vi "SA40060.20210626 BG.vi"() -> ()   [LabVIEW 2020]
uses:
  <vilib>/Analysis/baseanly.llb/Mean (DBL).vi
  <userlib>/_OpenG.lib/file/file.llb/Build Path - Traditional__ogtk.vi
  <userlib>/LevyLab/LV to ITX/Data/Data.lvclass
  <userlib>/LevyLab/XY Utilities/xy_utilities.lvlib
  <vilib>/Analysis/NI_AALBase.lvlib
panel:
  in  "Temps to keep (Lifespan)":i32=26
  out "Lifespan vs Temp (hrs)":cluster{i32[], dbl[]}[](graph)
  out "E_a":dbl[](array[numeric])
  out "Arrhenius":T1(graph)
  in  "Temps to keep (Arrhenius fit)":i32=26
  out "G2T vs t BG":T1(graph)
  out "G4T vs t BG":T1(graph)
  out "Temp vs t":T1(graph)
  in  "Source Voltage":dbl=0.1
  in  "Init Temp":i32=275
  in  "Temp Step":i32=5
  in  "Final Temp":i32=400
  in  "Data File":path=path "G:/My Drive/ansom/Data/PPMS 2/SA40060.20210626/00 - BG ONLY/SA40060.20210626.275K.dat"
  in  "Trimming":i32=400
  in  "Update":bool
  in  "OK":bool
  out "error out":errorcluster
  in  "error in (no error)":errorcluster
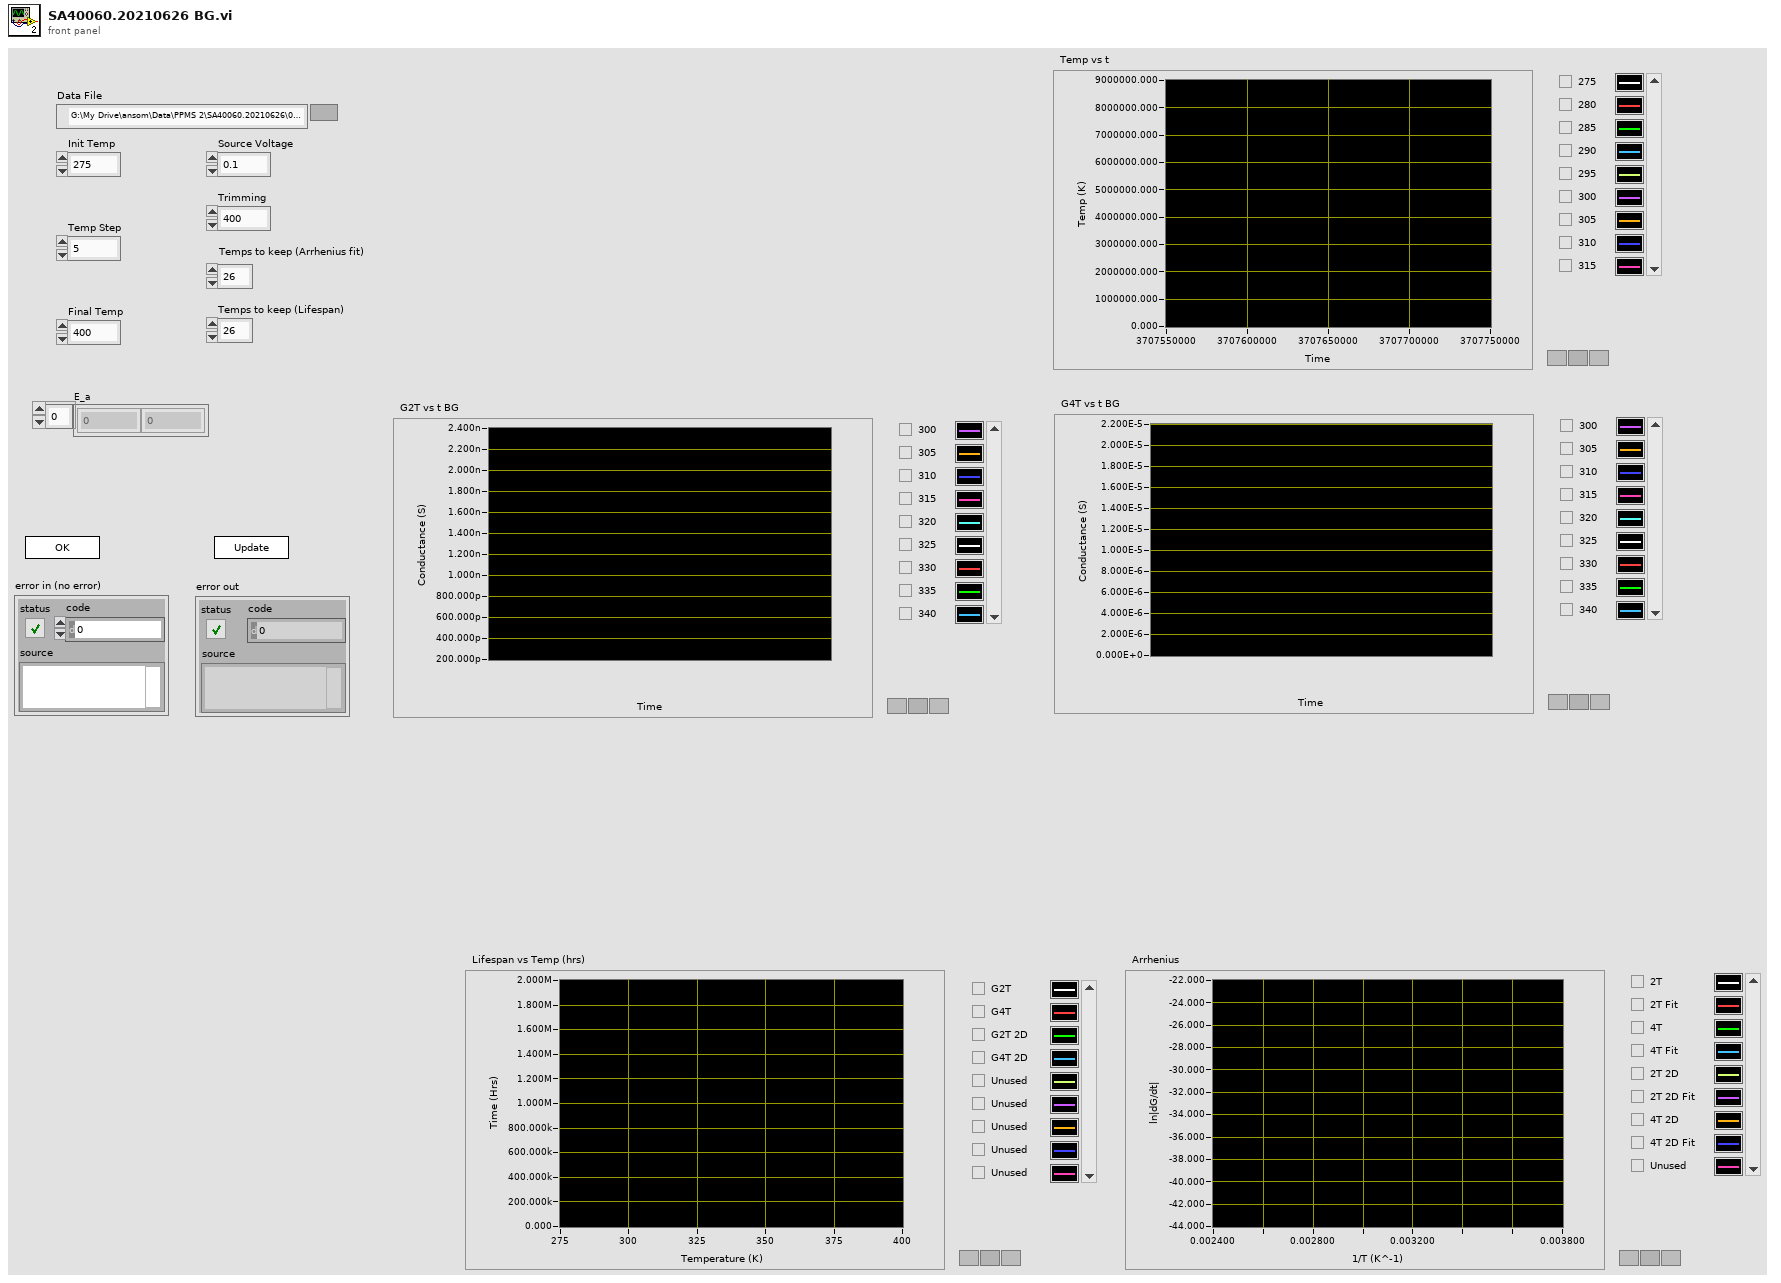
[diagram p1: front panel]
types:
  T1 = cluster{"Data":dbl[], "Best Exponential Fit":dbl[]}[]
  T2 = enum32{"Invalid", "Standard", "Closed", "Hidden", "Minimized", "Maximized"}
  T3 = enum32{"invalid app kind", "Development System", "Run Time System", "Student Edition", "Embedded LabVIEW", "Evaluation", "Custom"}
  T4 = cluster{"Core":cluster{"Current VI Reference":refnum<vi>, "Close Panel on Exit?":bool}, "G2T 1D":cluster{dbl[], dbl[]}[], "G4T 1D":cluster{dbl[], dbl[]}[], "Temp":cluster{dbl[], dbl[]}[], "Source Voltage":dbl, "Final Temp":i32, "Init Temp":i32, "Temp Step":i32, "Data File":path, "Trimming":i32}
  T5 = cluster{"Current VI Reference":refnum<vi>, "Close Panel on Exit?":bool}
  T6 = typedef "Data.lvclass/Dictionary--cluster.ctl" = cluster{"key":string, "value":variant}
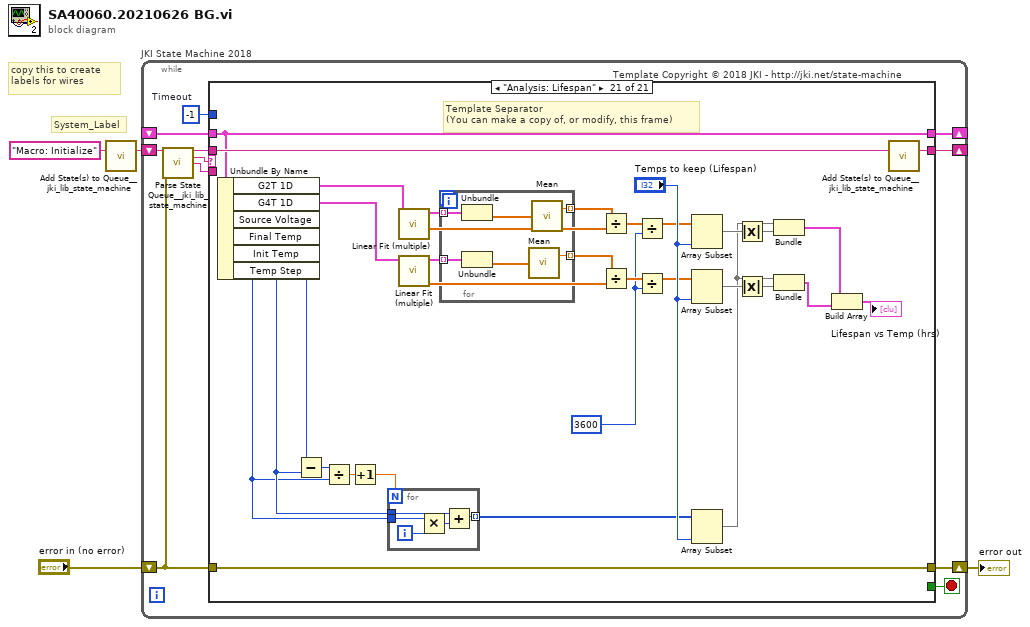
[diagram p0: block diagram]
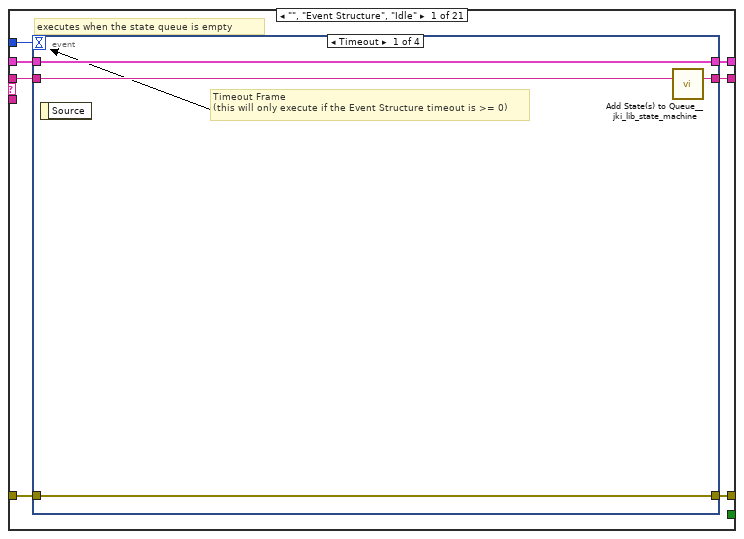
[diagram p2: hidden frame]
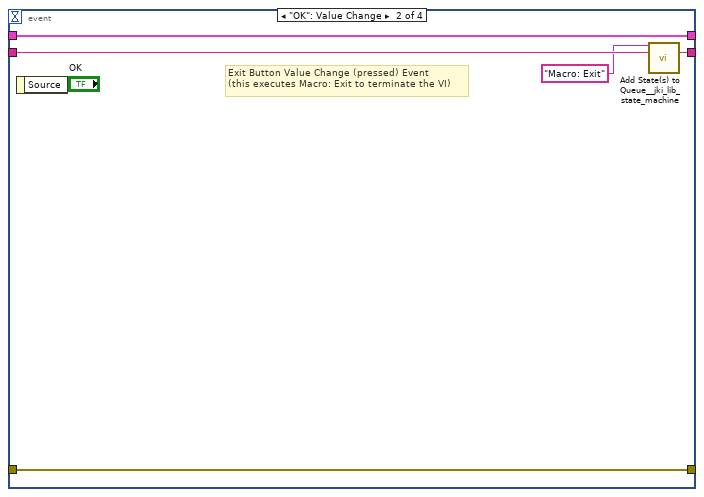
[diagram p3: hidden frame]
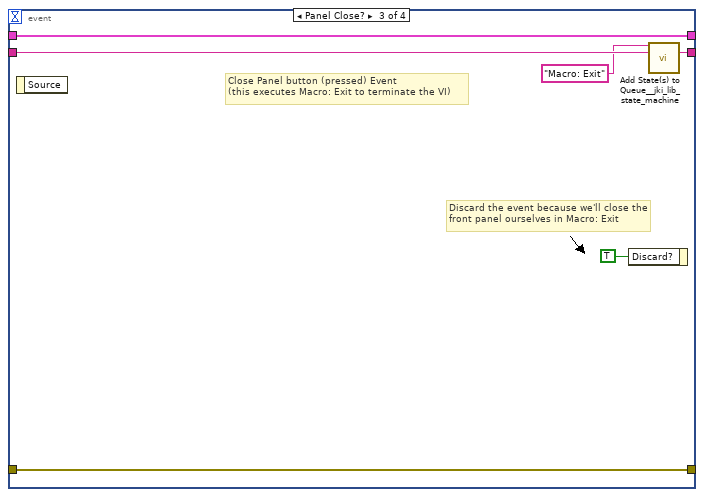
[diagram p4: hidden frame]
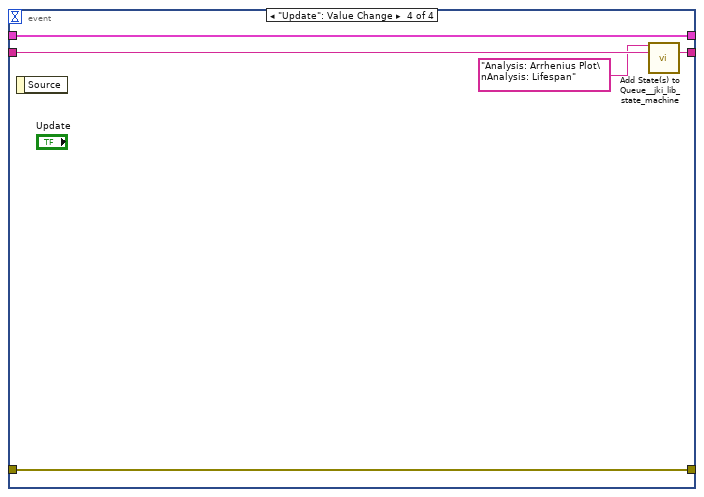
[diagram p5: hidden frame]
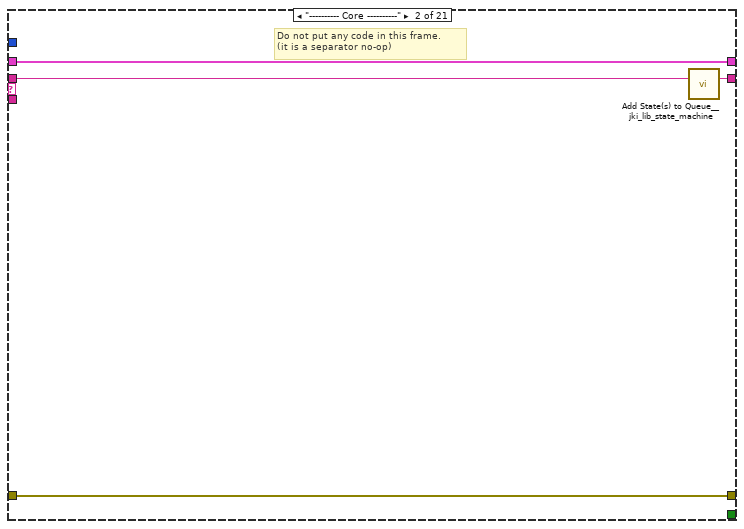
[diagram p6: hidden frame]
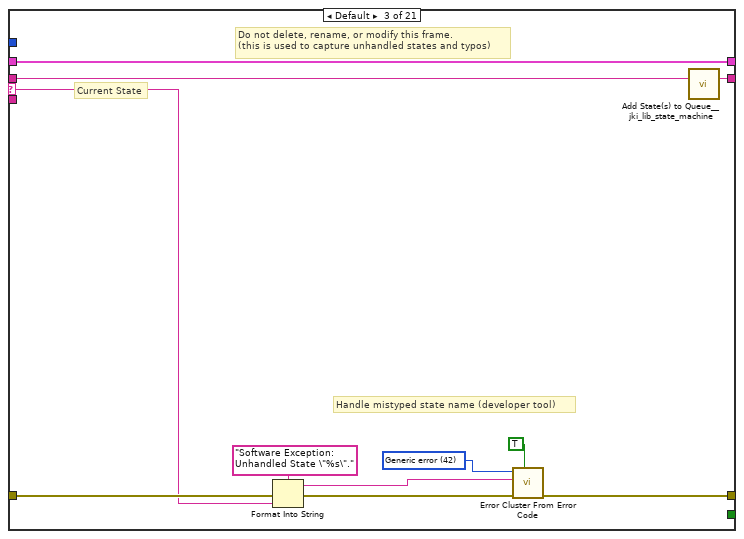
[diagram p7: hidden frame]
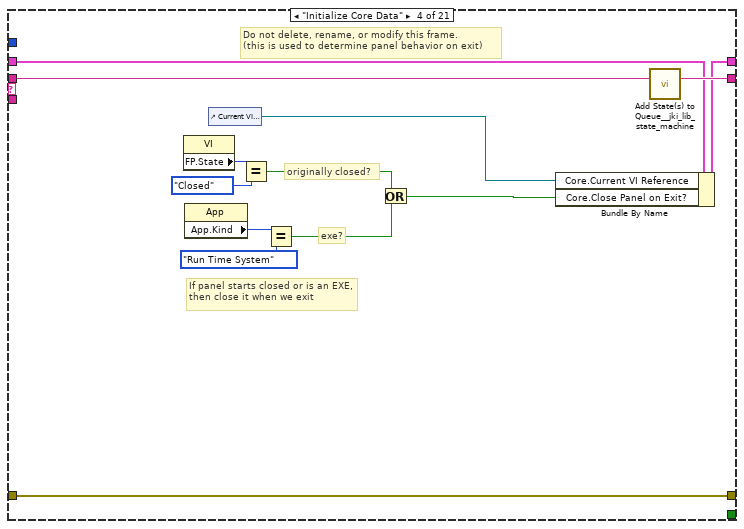
[diagram p8: hidden frame]
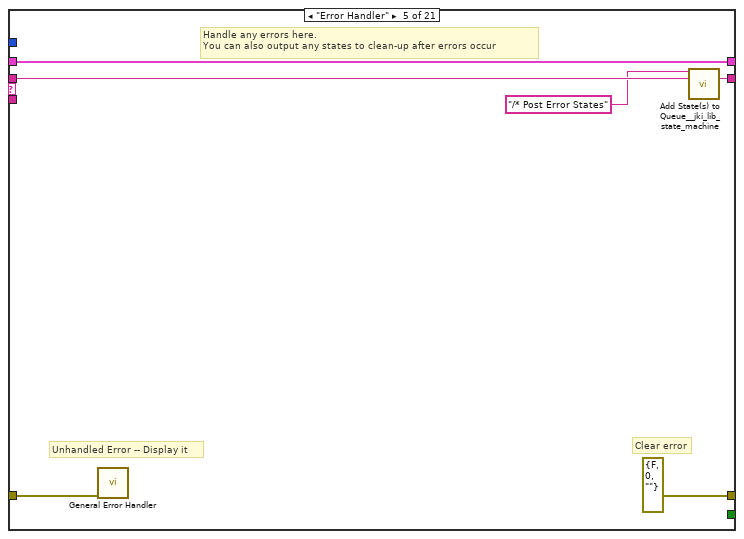
[diagram p9: hidden frame]
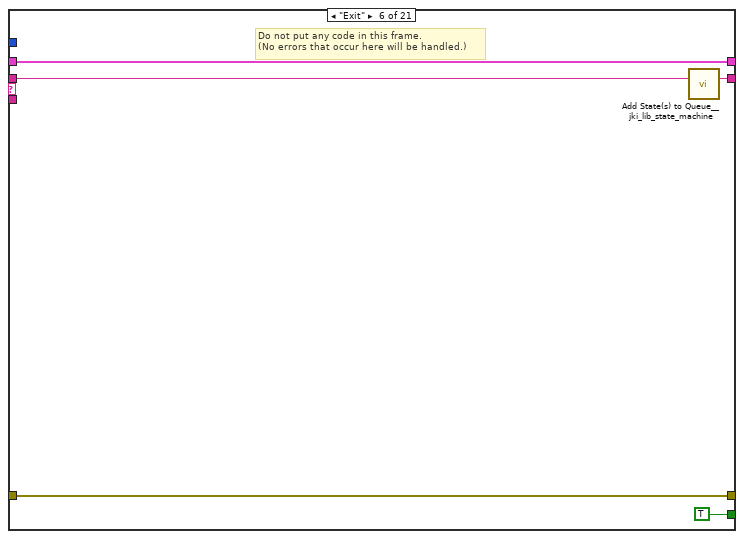
[diagram p10: hidden frame]
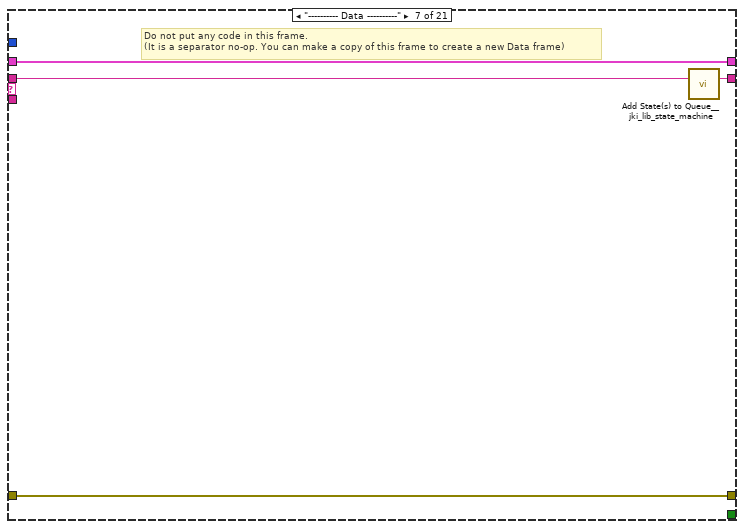
[diagram p11: hidden frame]
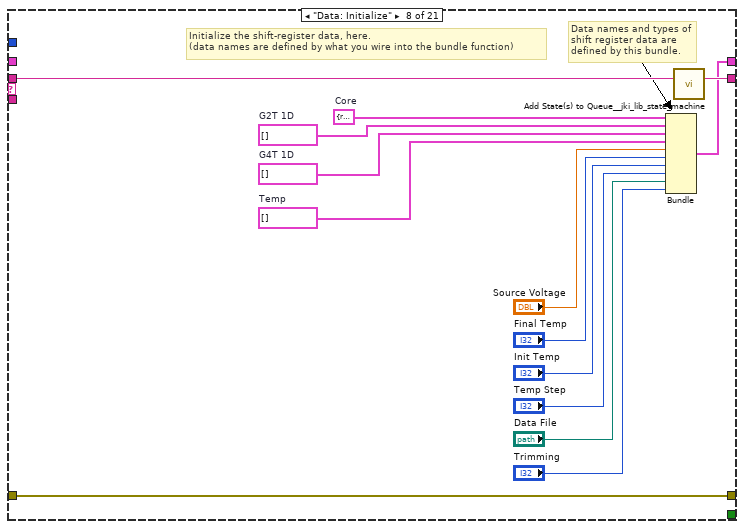
[diagram p12: hidden frame]
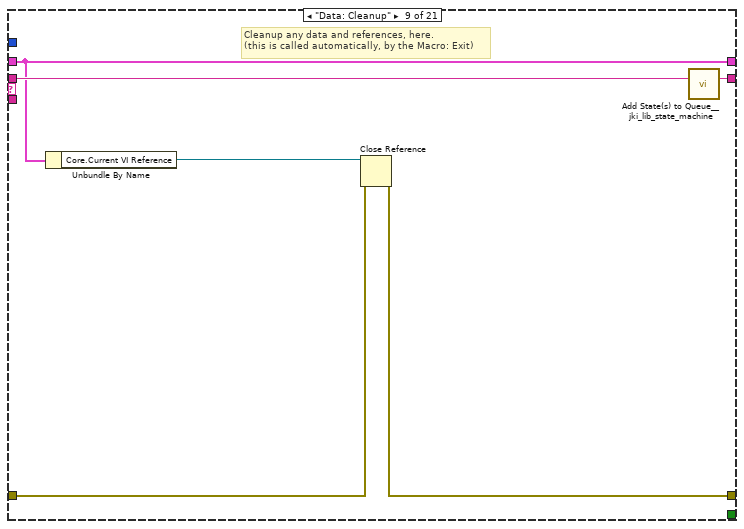
[diagram p13: hidden frame]
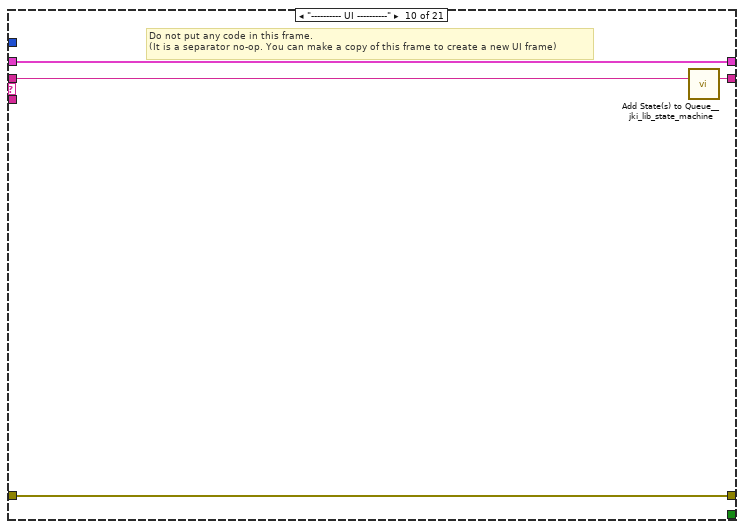
[diagram p14: hidden frame]
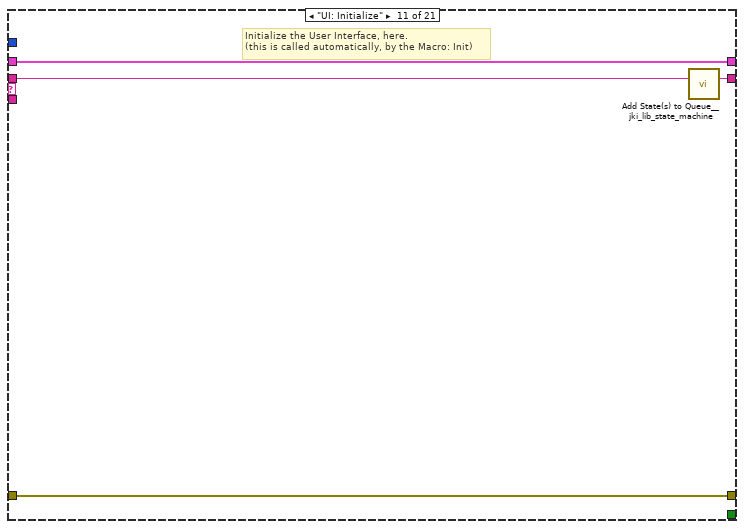
[diagram p15: hidden frame]
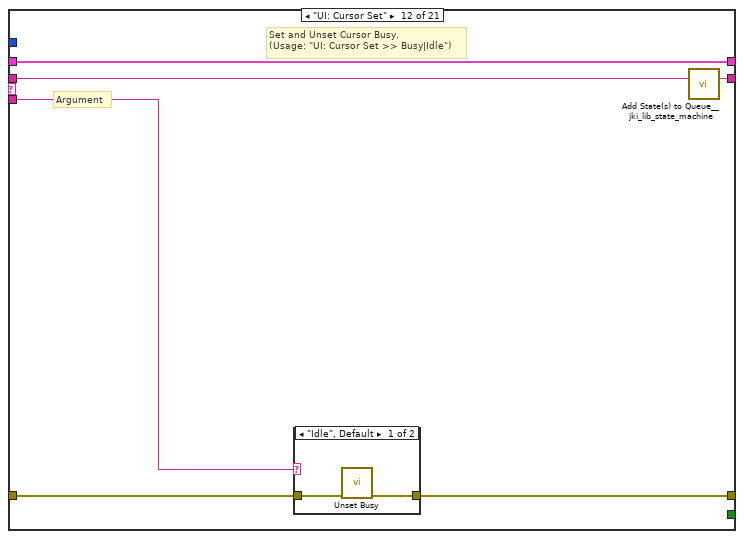
[diagram p16: hidden frame]
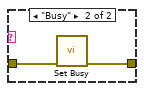
[diagram p17: hidden frame]
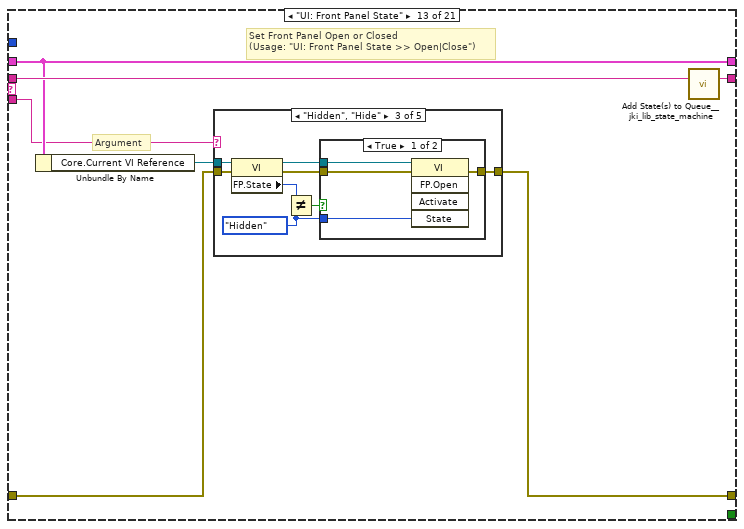
[diagram p18: hidden frame]
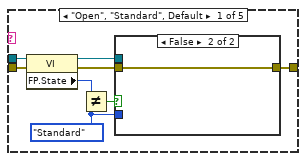
[diagram p19: hidden frame]
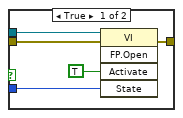
[diagram p20: hidden frame]
diagram:
  # "copy this to create labels for wires"
  # "System_Label"
  n1 = call <vilib>:"Add State(s) to Queue__jki_lib_state_machine.vi"("State(s) in (\"\")"="Macro: Initialize") -> ("States Out"=w4:string)  [unwired: 14 in]
  n2 = while "JKI State Machine 2018" {
    shift-right: [w8] -> _
    shift-left: _ -> [w7]
    shift-right: [w11] -> w1
    shift-left: "error in (no error)" -> [w5]
    shift-right: [w10] -> _
    shift-left: w4 -> [w12]
    stop <- w9 stop-if-true
    w6 = -1  # Timeout
    # "Template Copyright © 2018 JKI - http://jki.net/state-machine"
    n3 = call <vilib>:"Parse State Queue__jki_lib_state_machine.vi"("State Queue"=w12, "Error In (no error)"=w5) -> ("Remaining States"=w14:string, "Current State"=w15:string, "Arguments"=w13:string)  [unwired: 11 in]
    n4 = case shown="\"Analysis: Lifespan\"" w15 {
      selector: w15 -> [_ _ w47 _ _ _ _ _ _ _ _ _ _ _ _ _ _ _ _ _ _]
      tunnel: w14 -> [w22 w46 w51 w70 w76 w81 w85 w99 w105 w109 w113 w119 w130 w199 w204 w214 w218 w235 w282 w314 w353]
      tunnel: w13 -> [_ _ _ _ _ _ _ _ _ _ _ w114 w124 _ _ _ _ _ _ _ _]
      tunnel: w7 -> [w20 w43 w49 w63 w73 w79 w82 _ w100 w106 w111 w117 w126 w196 w201 w211 w215 w229 w279 w311 w339]
      tunnel: [w19 w44 w53 w67 errorcluster {"status"=FALSE, "code"=0, "source"=""} ("error out") w78 w83 w96 w101 w107 w110 w115 w127 w197 w202 w212 w216 w231 w280 w312 w351] -> w11
      tunnel: w5 -> [w18 w44 w52 w67 w72 w78 w83 w96 w102 w107 w110 w116 w128 w197 w202 w212 w216 w231 w280 w312 w351]
      tunnel: [w21 w45 w50 w69 w75 w80 w84 w98 w104 w108 w112 w118 w129 w198 w203 w213 w217 w234 w281 w313 w352] -> w10
      tunnel: [_ _ _ _ _ TRUE _ _ _ _ _ _ _ _ _ _ _ _ _ _ _] -> w9
      tunnel: [w17 w43 w49 w68 w73 w79 w82 w97 w100 w106 w111 w117 w126 w196 w201 w211 w215 w230 w279 w311 w339] -> w8
      tunnel: w6 -> [w16 _ _ _ _ _ _ _ _ _ _ _ _ _ _ _ _ _ _ _ _]
      frame "", "Event Structure", "Idle" {
        # "executes when the state queue is empty"
        n5 = event shown="[0] Timeout" {
          selector: _ -> [_ _ _ _]
          dyn-events: _ -> [_ _ _ _]
          timeout: w16 -> [_ _ _ _]
          tunnel: w22 -> [w26 w31 w37 w41]
          tunnel: [w25 w30 w36 w40] -> w21
          tunnel: w20 -> [w23 w28 w34 w42]
          tunnel: [w24 w29 w35 w38] -> w19
          tunnel: w18 -> [w24 w29 w35 w38]
          tunnel: [w23 w28 w34 w42] -> w17
          event Timeout {
            # "Timeout Frame\n(this will only execute if the Event Structure timeout is >= 0)"
            n6 = event-data() -> ()  [unwired: 1 in, 1 out]
            n7 = call <vilib>:"Add State(s) to Queue__jki_lib_state_machine.vi"("State(s) in (\"\")"=w26) -> ("States Out"=w25:string)  [unwired: 14 in]
          }
          event "OK": Value Change {
            # "Exit Button Value Change (pressed) Event\n(this executes Macro: Exit to terminate the VI)"
            n8 = event-data() -> ()  [unwired: 1 in, 1 out]
            n9 = call <vilib>:"Add State(s) to Queue__jki_lib_state_machine.vi"("State(s) in Front (\"\")"="Macro: Exit", "State(s) in (\"\")"=w31) -> ("States Out"=w30:string)  [unwired: 13 in]
          }
          event Panel Close? {
            # "Discard the event because we'll close the front panel ourselves in Macro: Exit"
            # "Close Panel button (pressed) Event\n(this executes Macro: Exit to terminate the VI)"
            n10 = event-data() -> ()  [unwired: 1 in, 1 out]
            n11 = event-data("Discard?"=TRUE) -> ()  [unwired: 1 in, 1 out]
            n12 = call <vilib>:"Add State(s) to Queue__jki_lib_state_machine.vi"("State(s) in Front (\"\")"="Macro: Exit", "State(s) in (\"\")"=w37) -> ("States Out"=w36:string)  [unwired: 13 in]
          }
          event "Update": Value Change {
            n13 = event-data() -> ()  [unwired: 1 in, 1 out]
            n14 = call <vilib>:"Add State(s) to Queue__jki_lib_state_machine.vi"("State(s) in Front (\"\")"="Analysis: Arrhenius Plot\nAnalysis: Lifespan" ("State(s) in Front (\"\")"), "State(s) in (\"\")"=w41) -> ("States Out"=w40:string)  [unwired: 13 in]
          }
        }
      }
      frame "---------- Core ----------" {
        # "Do not put any code in this frame.\n(it is a separator no-op)"
        n15 = call <vilib>:"Add State(s) to Queue__jki_lib_state_machine.vi"("State(s) in (\"\")"=w46) -> ("States Out"=w45:string)  [unwired: 14 in]
      }
      frame Default {
        w56 = 42 items=["No error", "Argument error", "Memory is full", "Out of zone", "End of file", "File already open", "Generic file I/O error", "File not found", "File permission error", "Disk is full", "Duplicate path", "Too many files open", "System feature not enabled", "Resource file not found", "Cannot add resource", "Resource not found", "Image not found", "Image memory error", "Pen does not exist", "Config type invalid", "Config token not found", "Config parse error", "Config memory error", "Bad external code format", "Bad external code offset", "External code not present", "Null window", "Destroy window error", "Null menu", "Print aborted", "Bad print record", "Print driver error", "Windows error during printing", "Memory error during printing", "Print dialog error", "Generic print error", "Invalid device refnum", "Device not found", "Device parameter error", "Device unit error", "Cannot open device", "Device call aborted", "Generic error", "Cancelled by user", "Object ID too low", "Object ID too high", "Object not in heap", "Unknown heap", "Unknown object (invalid DefProc)", "Unknown object (DefProc not in table)", "Message out of range", "Invalid (null) method", "Unknown message", "Manager call not supported", "Bad address", "Network operation in progress", "Network operation timed out", "Connection is busy", "Network attribute not supported", "Network error", "Address in use", "System out of memory", "Connection aborted", "Connection refused", "Not connected", "Already connected", "Connection closed", "Initialization error (interapplication manager)", "Bad occurrence", "Wait on unbound occurrence handler", "Occurrence queue overflow", "Datalog type conflict", "Unused", "Unrecognized type (interapplication manager)", "Memory corrupt", "Failed to make temporary DLL", "Old CIN version", "Drag socket not found", "Failed to load drop-object", "Failed to register OLE object", "Failed to release OLE object", "Format specifier type mismatch", "Unknown format specifier", "Too few format specifiers", "Too many format specifiers", "Scan failed", "Newer CIN version", "Error converting to variant", "Runtime menu error", "Password tampered", "Variant attribute not found", "Incompatible variant data type", "Event data is not available", "Event Store is not present", "Occurrence is not found", "Event Queue is not created", "Event info is not available", "Refnum passed is NULL", "Error retrieving Class GUID", "Error retrieving CoClass GUID", "Error retrieving TypeLib GUID.", "Bad built application magic bytes.", "Specific driver is different from the specific driver associated with the Logical Name.", "There is no session opened to the class driver.", "Max Error", "MAX - Error with config objects", "MAX - Error loading configuration", "MAX - Group not supported"]
        # "Current State"
        # "Do not delete, rename, or modify this frame.\n(this is used to capture unhandled states and typos)"
        # "Handle mistyped state name (developer tool)"
        n16 = Format Into String(format string="Software Exception: Unhandled State \"%s\"." ("message"), error in=w52, w47) -> (resulting string=w55:string, error out=w54:errorcluster)  [unwired: 1 in]
        n17 = call <vilib>:"Error Cluster From Error Code.vi"("show call chain? (False)"=TRUE, "error in (no error)"=w54, "error message (\"\")"=w55, "error code (0)"=w56) -> ("error out"=w53:errorcluster)  [unwired: 5 in]
        n18 = call <vilib>:"Add State(s) to Queue__jki_lib_state_machine.vi"("State(s) in (\"\")"=w51) -> ("States Out"=w50:string)  [unwired: 14 in]
      }
      frame "Initialize Core Data" {
        # "Do not delete, rename, or modify this frame.\n(this is used to determine panel behavior on exit)"
        # "originally closed?"
        # "exe?"
        # "If panel starts closed or is an EXE, then close it when we exit"
        n19 = property class="VI"() -> ("FP.State"=w60:T2)  [unwired: 2 in, 2 out]
        n20 = property class="App"() -> ("App.Kind"=w66:T3)  [unwired: 2 in, 2 out]
        n21 = control-ref of="Current VI Reference"() -> (w61:refnum<vi>)
        n22 = Equal?(x=w60, y=T2."Closed" ("Front Panel Window:State")) -> (x = y?=w58:bool)
        n23 = Equal?(x=w66, y=T3."Run Time System" ("Application:Kind")) -> (x = y?=w64:bool)
        n24 = Or(x=w58, y=w64) -> (x .or. y?=w62:bool)
        n25 = Bundle By Name(cluster=w63, "Core.Current VI Reference"=w61, "Core.Close Panel on Exit?"=w62) -> (w68:T4)
        n26 = call <vilib>:"Add State(s) to Queue__jki_lib_state_machine.vi"("State(s) in (\"\")"=w70) -> ("States Out"=w69:string)  [unwired: 14 in]
      }
      frame "Error Handler" {
        # "Unhandled Error -- Display it"
        # "Handle any errors here.\nYou can also output any states to clean-up after errors occur"
        # "Clear error"
        n27 = call <vilib>:"General Error Handler.vi"("error in (no error)"=w72) -> ()  [unwired: 10 in, 5 out]
        n28 = call <vilib>:"Add State(s) to Queue__jki_lib_state_machine.vi"("State(s) in Front (\"\")"="/* Post Error States", "State(s) in (\"\")"=w76) -> ("States Out"=w75:string)  [unwired: 13 in]
      }
      frame "Exit" {
        # "Do not put any code in this frame.\n(No errors that occur here will be handled.)"
        n29 = call <vilib>:"Add State(s) to Queue__jki_lib_state_machine.vi"("State(s) in (\"\")"=w81) -> ("States Out"=w80:string)  [unwired: 14 in]
      }
      frame "---------- Data ----------" {
        # "Do not put any code in this frame.\n(It is a separator no-op. You can make a copy of this frame to create a new Data frame)"
        n30 = call <vilib>:"Add State(s) to Queue__jki_lib_state_machine.vi"("State(s) in (\"\")"=w85) -> ("States Out"=w84:string)  [unwired: 14 in]
      }
      frame "Data: Initialize" {
        w86 = cluster{dbl[], dbl[]}[] []  # Temp
        w93 = cluster{dbl[], dbl[]}[] []  # G4T 1D
        w92 = cluster{dbl[], dbl[]}[] []  # G2T 1D
        w95 = T5 {"Current VI Reference"=refnum, "Close Panel on Exit?"=FALSE}  # Core
        # "Data names and types of shift register data are defined by this bundle."
        # "Initialize the shift-register data, here.\n(data names are defined by what you wire into the bundle function)"
        n31 = Bundle("Core"=w95, "G2T 1D"=w92, "G4T 1D"=w93, "Temp"=w86, "Source Voltage"="Source Voltage", "Final Temp"="Final Temp", "Init Temp"="Init Temp", "Temp Step"="Temp Step", "Data File"="Data File", "Trimming"="Trimming") -> (w97:T4)  [unwired: 1 in]
        n32 = call <vilib>:"Add State(s) to Queue__jki_lib_state_machine.vi"("State(s) in (\"\")"=w99) -> ("States Out"=w98:string)  [unwired: 14 in]
      }
      frame "Data: Cleanup" {
        # "Cleanup any data and references, here.\n(this is called automatically, by the Macro: Exit)"
        n33 = Unbundle By Name(w100) -> ("Core.Current VI Reference"=w103:refnum<vi>)
        n34 = Close Reference(reference=w103, error in (no error)=w102) -> (error out=w101:errorcluster)
        n35 = call <vilib>:"Add State(s) to Queue__jki_lib_state_machine.vi"("State(s) in (\"\")"=w105) -> ("States Out"=w104:string)  [unwired: 14 in]
      }
      frame "---------- UI ----------" {
        # "Do not put any code in this frame.\n(It is a separator no-op. You can make a copy of this frame to create a new UI frame)"
        n36 = call <vilib>:"Add State(s) to Queue__jki_lib_state_machine.vi"("State(s) in (\"\")"=w109) -> ("States Out"=w108:string)  [unwired: 14 in]
      }
      frame "UI: Initialize" {
        # "Initialize the User Interface, here.\n(this is called automatically, by the Macro: Init)"
        n37 = call <vilib>:"Add State(s) to Queue__jki_lib_state_machine.vi"("State(s) in (\"\")"=w113) -> ("States Out"=w112:string)  [unwired: 14 in]
      }
      frame "UI: Cursor Set" {
        # "Argument"
        # "Set and Unset Cursor Busy.\n(Usage: \"UI: Cursor Set >> Busy|Idle\")"
        n38 = case shown="\"Idle\", Default" w114 {
          tunnel: w116 -> [w121 w123]
          tunnel: [w120 w122] -> w115
          frame "Idle", Default {
            n39 = call <vilib>:"Unset Busy.vi"("error in (no error)"=w121) -> ("error out"=w120:errorcluster)  [unwired: 10 in]
          }
          frame "Busy" {
            n40 = call <vilib>:"Set Busy.vi"("error in (no error)"=w123) -> ("error out"=w122:errorcluster)  [unwired: 9 in, 1 out]
          }
        }
        n41 = call <vilib>:"Add State(s) to Queue__jki_lib_state_machine.vi"("State(s) in (\"\")"=w119) -> ("States Out"=w118:string)  [unwired: 14 in]
      }
      frame "UI: Front Panel State" {
        # "Argument"
        # "Set Front Panel Open or Closed\n(Usage: \"UI: Front Panel State >> Open|Close\")"
        n42 = Unbundle By Name(w126) -> ("Core.Current VI Reference"=w125:refnum<vi>)
        n43 = case shown="\"Hidden\", \"Hide\"" w124 {
          tunnel: w128 -> [w136 w151 w162 w175 w188]
          tunnel: [w138 w152 w164 w177 w190] -> w127
          tunnel: w125 -> [w137 w149 w163 w176 w189]
          frame "Open", "Standard", Default {
            w131 = T2."Standard" ("State")
            n44 = property class="VI"(reference=w137, error in=w136) -> (reference out=w134:refnum<vi>, error out=w135:errorcluster, "FP.State"=w133:T2)
            n45 = Not Equal?(x=w133, y=w131) -> (x != y?=w132:bool)
            n46 = case shown="False" w132 {
              tunnel: [w142 w144] -> w138
              tunnel: w135 -> [w141 w144]
              tunnel: w134 -> [w140 _]
              tunnel: w131 -> [w139 _]
              frame True {
                n47 = invoke class="VI" method="FP.Open"(reference=w140, error in=w141, "Activate"=TRUE, "State"=w139) -> (error out=w142:errorcluster)  [unwired: 1 in, 4 out]
              }
              frame False {
              }
            }
          }
          frame "Close", "Closed" {
            n48 = property class="VI"(reference=w149, error in=w151) -> (reference out=w148:refnum<vi>, error out=w150:errorcluster, "FP.State"=w146:T2)
            n49 = Not Equal?(x=w146, y=T2."Closed" ("Front Panel Window:State")) -> (x != y?=w145:bool)
            n50 = case shown="True" w145 {
              tunnel: [w153 w156] -> w152
              tunnel: w150 -> [w153 w155]
              tunnel: w148 -> [_ w154]
              frame False {
              }
              frame True {
                n51 = invoke class="VI" method="FP.Close"(reference=w154, error in=w155) -> (error out=w156:errorcluster)  [unwired: 1 in, 2 out]
              }
            }
          }
          frame "Hidden", "Hide" {
            w157 = T2."Hidden" ("State")
            n52 = property class="VI"(reference=w163, error in=w162) -> (reference out=w160:refnum<vi>, error out=w161:errorcluster, "FP.State"=w159:T2)
            n53 = Not Equal?(x=w159, y=w157) -> (x != y?=w158:bool)
            n54 = case shown="True" w158 {
              tunnel: [w168 w169] -> w164
              tunnel: w161 -> [w167 w169]
              tunnel: w160 -> [w166 _]
              tunnel: w157 -> [w165 _]
              frame True {
                n55 = invoke class="VI" method="FP.Open"(reference=w166, error in=w167, "State"=w165) -> (error out=w168:errorcluster)  [unwired: 2 in, 4 out]
              }
              frame False {
              }
            }
          }
          frame "Minimize", "Minimized" {
            w170 = T2."Minimized" ("State")
            n56 = property class="VI"(reference=w176, error in=w175) -> (reference out=w173:refnum<vi>, error out=w174:errorcluster, "FP.State"=w172:T2)
            n57 = Not Equal?(x=w172, y=w170) -> (x != y?=w171:bool)
            n58 = case shown="True" w171 {
              tunnel: [w181 w182] -> w177
              tunnel: w174 -> [w180 w182]
              tunnel: w173 -> [w179 _]
              tunnel: w170 -> [w178 _]
              frame True {
                n59 = invoke class="VI" method="FP.Open"(reference=w179, error in=w180, "State"=w178) -> (error out=w181:errorcluster)  [unwired: 2 in, 4 out]
              }
              frame False {
              }
            }
          }
          frame "Maximize", "Maximized" {
            w183 = T2."Maximized" ("State")
            n60 = property class="VI"(reference=w189, error in=w188) -> (reference out=w186:refnum<vi>, error out=w187:errorcluster, "FP.State"=w185:T2)
            n61 = Not Equal?(x=w185, y=w183) -> (x != y?=w184:bool)
            n62 = case shown="True" w184 {
              tunnel: [w194 w195] -> w190
              tunnel: w187 -> [w193 w195]
              tunnel: w186 -> [w192 _]
              tunnel: w183 -> [w191 _]
              frame True {
                n63 = invoke class="VI" method="FP.Open"(reference=w192, error in=w193, "State"=w191) -> (error out=w194:errorcluster)  [unwired: 2 in, 4 out]
              }
              frame False {
              }
            }
          }
        }
        n64 = call <vilib>:"Add State(s) to Queue__jki_lib_state_machine.vi"("State(s) in (\"\")"=w130) -> ("States Out"=w129:string)  [unwired: 14 in]
      }
      frame "---------- Macro ----------" {
        # "Do not put any code in this frame.\n(It is a separator no-op. You can make a copy of this frame to create a new Macro frame)"
        n65 = call <vilib>:"Add State(s) to Queue__jki_lib_state_machine.vi"("State(s) in (\"\")"=w199) -> ("States Out"=w198:string)  [unwired: 14 in]
      }
      frame "Macro: Initialize" {
        # "Initialization Macro\n(This is called once, when the VI starts)"
        n66 = call <vilib>:"Add State(s) to Queue__jki_lib_state_machine.vi"("State(s) in Front (\"\")"="Data: Initialize\nInitialize Core Data\nUI: Initialize\nUI: Front Panel State >> Open\nAnalysis: Load Data\nAnalysis: Plot G vs t\nAnalysis: Arrhenius Plot\nAnalysis: Lifespan", "State(s) in (\"\")"=w204) -> ("States Out"=w203:string)  [unwired: 13 in]
      }
      frame "Macro: Exit" {
        # "Exit Macro\n(This is called once, when the VI exits)"
        n67 = Unbundle By Name(w211) -> ("Core.Close Panel on Exit?"=w210:bool)
        n68 = Select(t="UI: Front Panel State >> Close", s=w210, f="") -> (s? t:f=w207:string)
        n69 = call <vilib>:"Add State(s) to Queue__jki_lib_state_machine.vi"("State(s) in (\"\")"=w207, "State(s) at Back (\"\")"="Data: Cleanup\nExit") -> ("States Out"=w205:string)  [unwired: 13 in]
        n70 = call <vilib>:"Add State(s) to Queue__jki_lib_state_machine.vi"("State(s) in Front (\"\")"=w205, "State(s) in (\"\")"=w214) -> ("States Out"=w213:string)  [unwired: 13 in]
      }
      frame "---------- Analysis ----------" {
        # "Template Separator\n(You can make a copy of, or modify, this frame)"
        n71 = call <vilib>:"Add State(s) to Queue__jki_lib_state_machine.vi"("State(s) in (\"\")"=w218) -> ("States Out"=w217:string)  [unwired: 14 in]
      }
      frame "Analysis: Load Data" {
        n72 = Unbundle By Name(w229) -> ("Source Voltage"=w228:dbl, "Final Temp"=w225:i32, "Init Temp"=w222:i32, "Temp Step"=w221:i32, "Data File"=w223:path, "Trimming"=w220:i32)
        n73 = Subtract(x=w225, y=w222) -> (x-y=w232:i32)
        n74 = Divide(x=w232, y=w221) -> (x/y=w233:dbl)
        n75 = Increment(x=w233) -> (x+1=w224:dbl)
        n76 = for {
          N: w224 -> [_]
          tunnel: w228 -> [w246]
          tunnel: [w263] -> w227 mode=indexing
          tunnel: [w262] -> w226 mode=indexing
          tunnel: w223 -> [w261]
          tunnel: w222 -> [w260]
          tunnel: w221 -> [w259]
          tunnel: w220 -> [w258]
          tunnel: [w255] -> w219 mode=indexing
          i -> [w266]
          n77 = Strip Path(path=w261) -> (stripped path=w271:path, name=w270:string)
          n78 = Multiply(x=w259, y=w266) -> (x*y=w267:i32)
          n79 = Add(x=w260, y=w267) -> (x+y=w272:i32)
          n80 = String Subset(string=w270, length (rest)=17) -> (substring=w268:string)  [unwired: 1 in]
          n81 = Format Into String(w272) -> (resulting string=w274:string)  [unwired: 3 in, 1 out]
          n82 = Concatenate Strings(w268, w274, "K.dat" ("string")) -> (w273:string)
          n83 = call-poly <userlib>:"Build Path__ogtk.vi"("name or relative path"=w273, "base path"=w271) -> ("appended path"=w275:path)
          n84 = call <userlib>:"Data Read.vi"("path"=w275) -> ("Data (Dictionary)"=w241:T6[])  [unwired: 7 in, 3 out]
          n85 = call "Read Dictionary.vi"("Numeric"=0, "Dictionary In"=w241) -> ("data"=w251:dbl[])
          n86 = call "Read Dictionary.vi"("Numeric"=10 ("index"), "Dictionary In"=w241) -> ("data"=w247:dbl[])
          n87 = call "Read Dictionary.vi"("Numeric"=5, "Dictionary In"=w241) -> ("data"=w239:dbl[])
          n88 = call "Read Dictionary.vi"("Numeric"=4, "Dictionary In"=w241) -> ("data"=w250:dbl[])
          n89 = call "Read Dictionary.vi"("Numeric"=1, "Dictionary In"=w241) -> ("data"=w249:dbl[])
          n90 = Array Subset(array=w239) -> (w238:dbl[])  [unwired: 2 in]
          n91 = Array Subset(array=w251, index=w258) -> (w257:dbl[])  [unwired: 1 in]
          n92 = Array Subset(array=w247, index=w258) -> (w245:dbl[])  [unwired: 1 in]
          n93 = Array Subset(array=w250, index=w258) -> (w237:dbl[])  [unwired: 1 in]
          n94 = Subtract(x=w238, y=w237) -> (x-y=w236:dbl[])
          n95 = Divide(x=w245, y=w246) -> (x/y=w265:dbl[])
          n96 = Absolute Value(x=w265) -> (abs(x)=w244:dbl[])
          n97 = Array Subset(array=w249) -> (w256:dbl[])  [unwired: 2 in]
          n98 = Divide(x=w245, y=w236) -> (x/y=w242:dbl[])
          n99 = Bundle(w257, w244) -> (w263:cluster{dbl[], dbl[]})  [unwired: 1 in]
          n100 = Bundle(w257, w256) -> (w255:cluster{dbl[], dbl[]})  [unwired: 1 in]
          n101 = Absolute Value(x=w242) -> (abs(x)=w243:dbl[])
          n102 = Bundle(w257, w243) -> (w262:cluster{dbl[], dbl[]})  [unwired: 1 in]
        }
        n103 = call <vilib>:"Add State(s) to Queue__jki_lib_state_machine.vi"("State(s) in (\"\")"=w235) -> ("States Out"=w234:string)  [unwired: 14 in]
        n104 = Bundle By Name(cluster=w229, "G2T 1D"=w227, "G4T 1D"=w226, "Temp"=w219) -> (w230:T4)
      }
      frame "Analysis: Plot G vs t" {
        n105 = Unbundle By Name(w279) -> ("G2T 1D"=→"G2T vs t BG":cluster{dbl[], dbl[]}[], "G4T 1D"=→"G4T vs t BG":cluster{dbl[], dbl[]}[], "Temp"=→"Temp vs t":cluster{dbl[], dbl[]}[])
        n106 = call <vilib>:"Add State(s) to Queue__jki_lib_state_machine.vi"("State(s) in (\"\")"=w282) -> ("States Out"=w281:string)  [unwired: 14 in]
      }
      frame "Analysis: Arrhenius Plot" {
        n107 = Unbundle By Name(w311) -> ("G2T 1D"=w286:cluster{dbl[], dbl[]}[], "G4T 1D"=w285:cluster{dbl[], dbl[]}[], "Final Temp"=w308:i32, "Init Temp"=w306:i32, "Temp Step"=w305:i32)  [unwired: 1 out]
        n108 = Subtract(x=w308, y=w306) -> (x-y=w309:i32)
        n109 = Divide(x=w309, y=w305) -> (x/y=w310:dbl)
        n110 = Increment(x=w310) -> (x+1=w307:dbl)
        n111 = for {
          N: w307 -> [_]
          tunnel: w306 -> [w317]
          tunnel: w305 -> [w318]
          tunnel: [w315] -> w297 mode=indexing
          i -> [w319]
          n112 = Multiply(x=w318, y=w319) -> (x*y=w320:i32)
          n113 = Add(x=w317, y=w320) -> (x+y=w316:i32)
          n114 = Reciprocal(x=w316) -> (1/x=w315:dbl)
        }
        n115 = call-poly <userlib>:"Linear Fit.vi"("XY-data"=w286) -> ("slopes"=w283:dbl[])  [unwired: 4 in, 6 out]
        n116 = call-poly <userlib>:"Linear Fit.vi"("XY-data"=w285) -> ("slopes"=w284:dbl[])  [unwired: 4 in, 6 out]
        n117 = Absolute Value(x=w283) -> (abs(x)=w303:dbl[])
        n118 = Absolute Value(x=w284) -> (abs(x)=w304:dbl[])
        n119 = Natural Logarithm(1:w303) -> (0:w299:dbl[])
        n120 = Natural Logarithm(1:w304) -> (0:w298:dbl[])
        n121 = Array Subset(array=w299, length="Temps to keep (Arrhenius fit)") -> (w295:dbl[])  [unwired: 1 in]
        n122 = Array Subset(array=w298, length="Temps to keep (Arrhenius fit)") -> (w294:dbl[])  [unwired: 1 in]
        n123 = Array Subset(array=w297, length="Temps to keep (Arrhenius fit)") -> (w293:dbl[])  [unwired: 1 in]
        n124 = Bundle(w293, w295) -> (w301:cluster{dbl[], dbl[]})  [unwired: 1 in]
        n125 = Bundle(w293, w294) -> (w302:cluster{dbl[], dbl[]})  [unwired: 1 in]
        n126 = Build Array(w301, w302) -> (w290:cluster{dbl[], dbl[]}[])
        n127 = call-poly <userlib>:"Linear Fit.vi"("XY-data"=w290) -> ("Best Fits"=w289:cluster{"X-array":dbl[], "Y-array":dbl[]}[], "XY-data out"=w288:cluster{"X-array":dbl[], "Y-array":dbl[]}[], "slopes"=w287:dbl[])  [unwired: 4 in, 4 out]
        n128 = Multiply(x=w287, y=8.617333e-05) -> (x*y=→"E_a":dbl[])
        n129 = Interleave 1D Arrays(w288, w289) -> (→"Arrhenius":cluster{"X-array":dbl[], "Y-array":dbl[]}[])
        n130 = call <vilib>:"Add State(s) to Queue__jki_lib_state_machine.vi"("State(s) in (\"\")"=w314) -> ("States Out"=w313:string)  [unwired: 14 in]
      }
      frame "Analysis: Lifespan" {
        w325 = 3600
        # "Template Separator\n(You can make a copy of, or modify, this frame)"
        n131 = Unbundle By Name(w339) -> ("G2T 1D"=w350:cluster{dbl[], dbl[]}[], "G4T 1D"=w349:cluster{dbl[], dbl[]}[], "Final Temp"=w346:i32, "Init Temp"=w338:i32, "Temp Step"=w337:i32)  [unwired: 1 out]
        n132 = Subtract(x=w346, y=w338) -> (x-y=w347:i32)
        n133 = Divide(x=w347, y=w337) -> (x/y=w348:dbl)
        n134 = Increment(x=w348) -> (x+1=w336:dbl)
        n135 = for {
          N: w336 -> [_]
          tunnel: w338 -> [w362]
          tunnel: w337 -> [w361]
          tunnel: [w360] -> w335 mode=indexing
          i -> [w363]
          n136 = Multiply(x=w361, y=w363) -> (x*y=w364:i32)
          n137 = Add(x=w362, y=w364) -> (x+y=w360:i32)
        }
        n138 = call <userlib>:"Linear Fit (multiple).vi"("XY-data"=w350) -> ("XY-data out"=w332:cluster{"X-array":dbl[], "Y-array":dbl[]}[], "slopes"=w334:dbl[])  [unwired: 4 in, 5 out]
        n139 = call <userlib>:"Linear Fit (multiple).vi"("XY-data"=w349) -> ("XY-data out"=w331:cluster{"X-array":dbl[], "Y-array":dbl[]}[], "slopes"=w333:dbl[])  [unwired: 4 in, 5 out]
        n140 = for {
          tunnel: w332 -> [w358] mode=indexing
          tunnel: w331 -> [w359] mode=indexing
          tunnel: [w355] -> w330 mode=indexing
          tunnel: [w354] -> w329 mode=indexing
          n141 = Unbundle(w358) -> ("Y-array"=w356:dbl[])  [unwired: 1 out]
          n142 = Unbundle(w359) -> ("Y-array"=w357:dbl[])  [unwired: 1 out]
          n143 = call-poly <vilib>:"Mean.vi"("X"=w357) -> ("mean"=w354:dbl)  [unwired: 1 out]
          n144 = call-poly <vilib>:"Mean.vi"("X"=w356) -> ("mean"=w355:dbl)  [unwired: 1 out]
        }
        n145 = Divide(x=w330, y=w334) -> (x/y=w327:dbl[])
        n146 = Divide(x=w329, y=w333) -> (x/y=w326:dbl[])
        n147 = Divide(x=w327, y=w325) -> (x/y=w323:dbl[])
        n148 = Divide(x=w326, y=w325) -> (x/y=w324:dbl[])
        n149 = Array Subset(array=w323, length="Temps to keep (Lifespan)") -> (w342:dbl[])  [unwired: 1 in]
        n150 = Array Subset(array=w324, length="Temps to keep (Lifespan)") -> (w341:dbl[])  [unwired: 1 in]
        n151 = Array Subset(array=w335, length="Temps to keep (Lifespan)") -> (w340:i32[])  [unwired: 1 in]
        n152 = Absolute Value(x=w342) -> (abs(x)=w321:dbl[])
        n153 = Absolute Value(x=w341) -> (abs(x)=w322:dbl[])
        n154 = Bundle(w340, w321) -> (w344:cluster{i32[], dbl[]})  [unwired: 1 in]
        n155 = Bundle(w340, w322) -> (w345:cluster{i32[], dbl[]})  [unwired: 1 in]
        n156 = Build Array(w344, w345) -> (→"Lifespan vs Temp (hrs)":cluster{i32[], dbl[]}[])
        n157 = call <vilib>:"Add State(s) to Queue__jki_lib_state_machine.vi"("State(s) in (\"\")"=w353) -> ("States Out"=w352:string)  [unwired: 14 in]
      }
    }
  }
  "error out" <- w1
